vi "Waveform Data Averager.vi"(6 "uS Low":dbl, 7 "Samples Per Average":i32, 10 "V to uS Conversion":dbl, 11 "Voltage Array In":dbl[](array[numeric])) -> (2 "uS Array Out":dbl[](array[numeric]), 3 "Voltage Array Out":dbl[](array[numeric]))   [LabVIEW 2016]
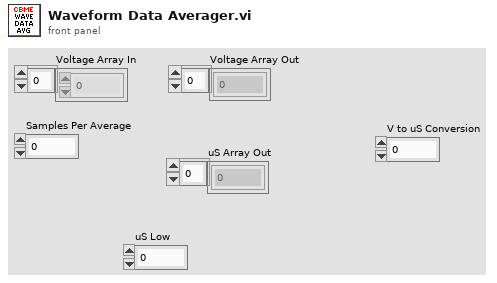
[diagram p1: front panel]
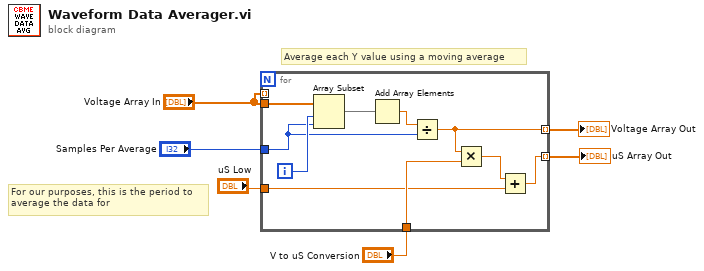
[diagram p0: block diagram]
diagram:
  # "Average each Y value using a moving average"
  # "For our purposes, this is the period to\naverage the data for"
  n1 = for {
    tunnel: "Voltage Array In" -> [_] mode=indexing
    tunnel: "Voltage Array In" -> [w16]
    tunnel: "Samples Per Average" -> [w12]
    tunnel: [w11] -> w6 mode=indexing
    tunnel: "V to uS Conversion" -> [w10]
    tunnel: [w8] -> w2 mode=indexing
    tunnel: "uS Low" -> [w7]
    i -> [w15]
    n2 = Array Subset(array=w16, index=w15, length=w12) -> (w14:dbl[])
    n3 = Add Array Elements(numeric array=w14) -> (sum=w13:dbl)
    n4 = Divide(x=w13, y=w12) -> (x/y=w11:dbl)
    n5 = Multiply(x=w11, y=w10) -> (x*y=w9:dbl)
    n6 = Add(x=w9, y=w7) -> (x+y=w8:dbl)
  }
  "Voltage Array Out" <- w6
  "uS Array Out" <- w2
